vi "Create Label Text.vi"(0 "Tick Cluster Array":T1, 1 "Reverse?":bool, 2 "Right justified":bool, 3 "Label Object Name":string, 5 "Range":cluster{"Max":sgl, "Min":sgl}, 7 "Alpha":sgl, 9 "Width":sgl, 11 "error in (no error)":errorcluster, 12 "Draw Last Label?":bool=TRUE, 13 "Draw First Label?":bool=TRUE, 14 "Color Box":u32(colorbox)) -> (4 "New Label Object":refnum<vi>, 8 "Max Width":sgl, 15 "error out":errorcluster)   [LabVIEW 2017, in "3D Plot.lvclass"]
uses:
  <vilib>/Math Plots/3D Math Plots/3D Plot/3D Plot/3D Plot.lvclass
  <vilib>/Math Plots/3D Math Plots/3D Plot/3D Plot/Typedef/Tick Array.ctl
  <vilib>/picture/3D Picture Control/Object/Create Object (name).vi
  <vilib>/picture/3D Picture Control/NI_3D Picture Control.lvlib
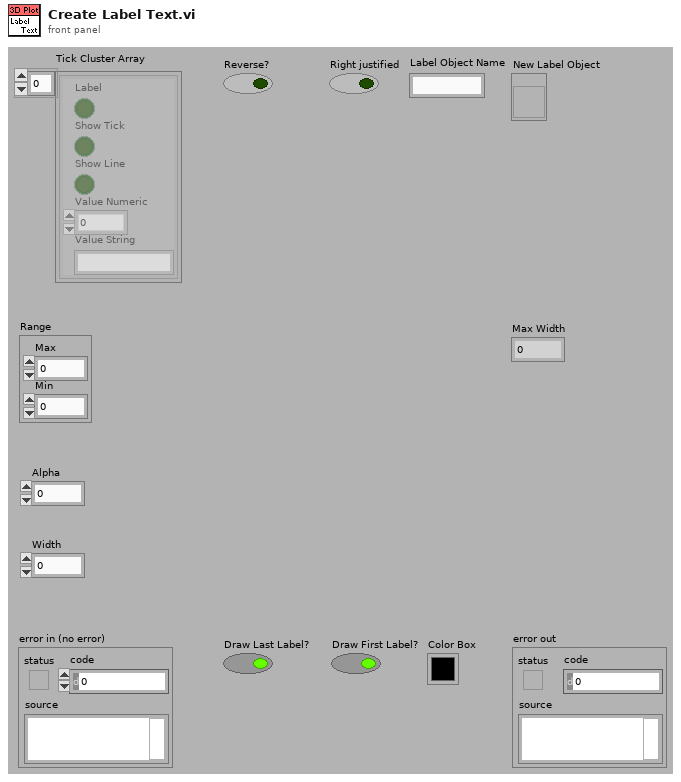
[diagram p1: front panel]
types:
  T1 = typedef "3D Plot.lvclass/Tick Array.ctl" = cluster{"Label":bool, "Show Tick":bool, "Show Line":bool, "Value Numeric":sgl, "Value String":string}[]
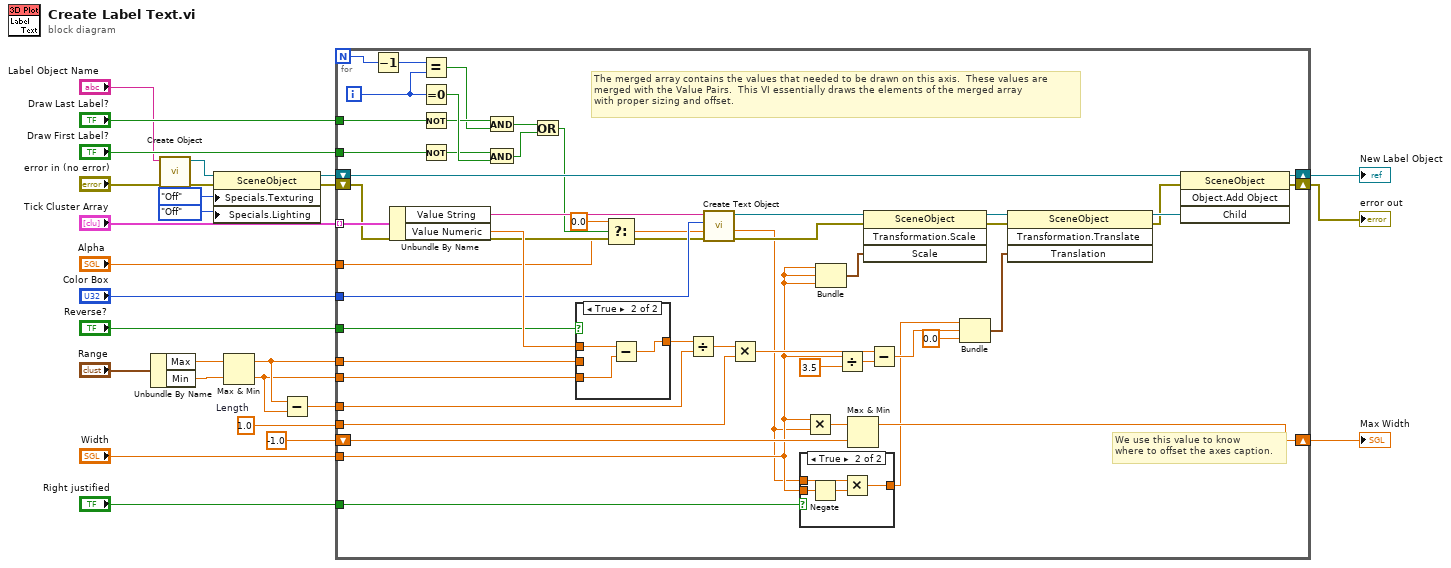
[diagram p0: block diagram]
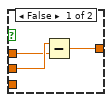
[diagram p2: hidden frame]
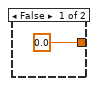
[diagram p3: hidden frame]
diagram:
  w2 = sgl 1.0  # Length
  n1 = Unbundle By Name("Range") -> ("Max"=w7:sgl, "Min"=w6:sgl)
  n2 = call-poly <vilib>:"Create Object.vi"("error in (no error)"="error in (no error)", "Name"="Label Object Name") -> ("error out"=w5:errorcluster, "Scene:New Object"=w12:refnum<vi>)  [unwired: 8 in]
  n3 = property class="SceneObject"(reference=w12, error in=w5, "Specials.Texturing"=enum16{"Inherit Value", "Off", "On"}."Off" ("Specials:Texturing"), "Specials.Lighting"=enum16{"Inherit Value", "Off", "On"}."Off" ("Specials:Lighting")) -> (reference out=w4:refnum<vi>, error out=w3:errorcluster)
  n4 = Max & Min(x=w7, y=w6) -> (max(x,y)=w10:sgl, min(x,y)=w9:sgl)
  n5 = Subtract(x=w10, y=w9) -> (x-y=w8:sgl)
  n6 = for {
    N -> [w54]
    tunnel: w2 -> [w70]
    tunnel: "Width" -> [w41]
    shift-right: [w73] -> w26
    shift-left: sgl -1.0 -> [w74]
    tunnel: "Tick Cluster Array" -> [w68] mode=indexing
    tunnel: w10 -> [w64]
    tunnel: w9 -> [w62]
    tunnel: w8 -> [w71]
    tunnel: "Reverse?" -> [w61]
    tunnel: "Right justified" -> [w48]
    tunnel: "Color Box" -> [w47]
    tunnel: "Draw First Label?" -> [w43]
    tunnel: "Draw Last Label?" -> [w42]
    shift-right: [w38] -> w19
    shift-left: w4 -> [w77]
    shift-right: [w34] -> w18
    shift-left: w3 -> [w33]
    tunnel: "Alpha" -> [w28]
    i -> [w53]
    # "The merged array contains the values that needed to be drawn on this axis.  These values are\nmerged with the Value Pairs.  This VI essentially draws the elements of the merged array\nwith proper sizing and offset."
    # "We use this value to know\nwhere to offset the axes caption."
    n7 = Decrement(x=w54) -> (x-1=w55:i32)
    n8 = Unbundle By Name(w68) -> ("Value String"=w67:string, "Value Numeric"=w63:sgl)
    n9 = Equal?(x=w55, y=w53) -> (x = y?=w51:bool)
    n10 = Equal To 0?(x=w53) -> (x = 0?=w60:bool)
    n11 = Not(x=w42) -> (.not. x?=w52:bool)
    n12 = Not(x=w43) -> (.not. x?=w59:bool)
    n13 = And(x=w52, y=w51) -> (x .and. y?=w50:bool)
    n14 = And(x=w59, y=w60) -> (x .and. y?=w49:bool)
    n15 = Or(x=w50, y=w49) -> (x .or. y?=w31:bool)
    n16 = case shown="True" w61 {
      tunnel: [w80 w81] -> w66
      tunnel: w64 -> [w79 _]
      tunnel: w63 -> [w78 w83]
      tunnel: w62 -> [_ w82]
      frame False {
        n17 = Subtract(x=w79, y=w78) -> (x-y=w80:sgl)
      }
      frame True {
        n18 = Subtract(x=w83, y=w82) -> (x-y=w81:sgl)
      }
    }
    n19 = Select(t=sgl 0.0, s=w31, f=w28) -> (s? t:f=w29:sgl)
    n20 = Divide(x=w66, y=w71) -> (x/y=w69:sgl)
    n21 = call <vilib>:"Create Text Object.vi"("error in (no error)"=w33, "Alpha"=w29, "Color Box"=w47, "Value String"=w67) -> ("error out"=w37:errorcluster, "Numeric"=w32:sgl, "Scene:New Object"=w44:refnum<vi>)  [unwired: 5 out]
    n22 = Multiply(x=w69, y=w70) -> (x*y=w65:sgl)
    n23 = case shown="True" w48 {
      tunnel: w41 -> [_ w88]
      tunnel: [sgl 0.0 w87] -> w39
      tunnel: w32 -> [_ w86]
      frame False {
      }
      frame True {
        n24 = Negate(x=w88) -> (-x=w85:sgl)
        n25 = Multiply(x=w86, y=w85) -> (x*y=w87:sgl)
      }
    }
    n26 = Multiply(x=w41, y=w32) -> (x*y=w72:sgl)
    n27 = Bundle("Width"=w41, "Width"=w41, "Width"=w41) -> (w75:cluster{"Width":sgl, "Width":sgl, "Width":sgl})  [unwired: 1 out]
    n28 = Divide(x=w41, y=sgl 3.5) -> (x/y=w57:sgl)
    n29 = Max & Min(x=w72, y=w74) -> (max(x,y)=w73:sgl)  [unwired: 1 out]
    n30 = invoke class="SceneObject" method="Transformation.Scale"(reference=w44, error in=w37, "Scale"=w75) -> (reference out=w45:refnum<vi>, error out=w36:errorcluster)  [unwired: 1 in, 2 out]
    n31 = Subtract(x=w65, y=w57) -> (x-y=w58:sgl)
    n32 = Bundle(w39, w58, "Y"=sgl 0.0) -> (w76:cluster{sgl, sgl, "Y":sgl})  [unwired: 1 out]
    n33 = invoke class="SceneObject" method="Transformation.Translate"(reference=w45, error in=w36, "Translation"=w76) -> (reference out=w46:refnum<vi>, error out=w35:errorcluster)  [unwired: 1 in, 2 out]
    n34 = invoke class="SceneObject" method="Object.Add Object"(reference=w77, error in=w35, "Child"=w46) -> (reference out=w38:refnum<vi>, error out=w34:errorcluster)  [unwired: 1 in, 2 out]
  }
  "error out" <- w18
  "Max Width" <- w26
  "New Label Object" <- w19
